vi "DMS_Insert.vi"(4 "Serial No":i32, 7 "DMS":T2, 8 "error in (no error)":errorcluster, 9 "Machine Code":string, 11 "Ref in":T4={"MS SQL Connection"=refnum, "UDL File"=path "", "Time"="", "DCODE"="", "WIP+1"=0, "MC No?"=0, "POKAYOKE?"=FALSE, "Expected Result"="", "Result [Status]"="", "Clock"=0.0, "RFID"="", "WIP Queue"=refnum, "TS Parameter"={"ProfitCenterCode"="", "LineCode"="", "WorkOrderNumber"="", "Model"="", "Model_with_Prefix"="", "VendorCode"="", "SetParameterDateCode"="", "PokaYoke"=0, "Target"=1, "Live_DateCode"="", "CustomerPartNumber"="", "Hand"="", "sBarcode"=FALSE, "FCA"=0, "Ent_Stamp"=timestamp(0 s since 1904-01-01), "STS_CD"=0.0}, "Data_Queue"=[], "RFID Serial No."=""} {"TS Parameter"."FCA" format="%01d"; "TS Parameter"."Target" min=1 max=100000; "TS Parameter"."PokaYoke" min=0 max=1}) -> (0 "error out":errorcluster, 1 "Message":string, 3 "Ref Out":T4={"MS SQL Connection"=refnum, "UDL File"=path "", "Time"="", "DCODE"="", "WIP+1"=0, "MC No?"=0, "POKAYOKE?"=FALSE, "Expected Result"="", "Result [Status]"="", "Clock"=0.0, "RFID"="", "WIP Queue"=refnum, "TS Parameter"={"ProfitCenterCode"="", "LineCode"="", "WorkOrderNumber"="", "Model"="", "Model_with_Prefix"="", "VendorCode"="", "SetParameterDateCode"="", "PokaYoke"=0, "Target"=1, "Live_DateCode"="", "CustomerPartNumber"="", "Hand"="", "sBarcode"=FALSE, "FCA"=0, "Ent_Stamp"=timestamp(0 s since 1904-01-01), "STS_CD"=0.0}, "Data_Queue"=[], "RFID Serial No."=""} {"TS Parameter"."FCA" format="%01d"; "TS Parameter"."Target" min=1 max=100000; "TS Parameter"."PokaYoke" min=0 max=1})   [LabVIEW 2020]
uses:
  Controls/TD SQL.ctl
  <vilib>/addons/database/Connection.llb/Conn ObjectReference.ctl
  Controls/WIP_State.ctl
  Controls/TS_Parameter.ctl
  Controls/DMS_Control.ctl
  Controls/dms_BOOL.ctl
  MS SQL/MS_Global.vi
  <vilib>/addons/database/NI_Database_API.lvlib
panel:
  in  "Machine":T1(ring)
  out "resulting string":string
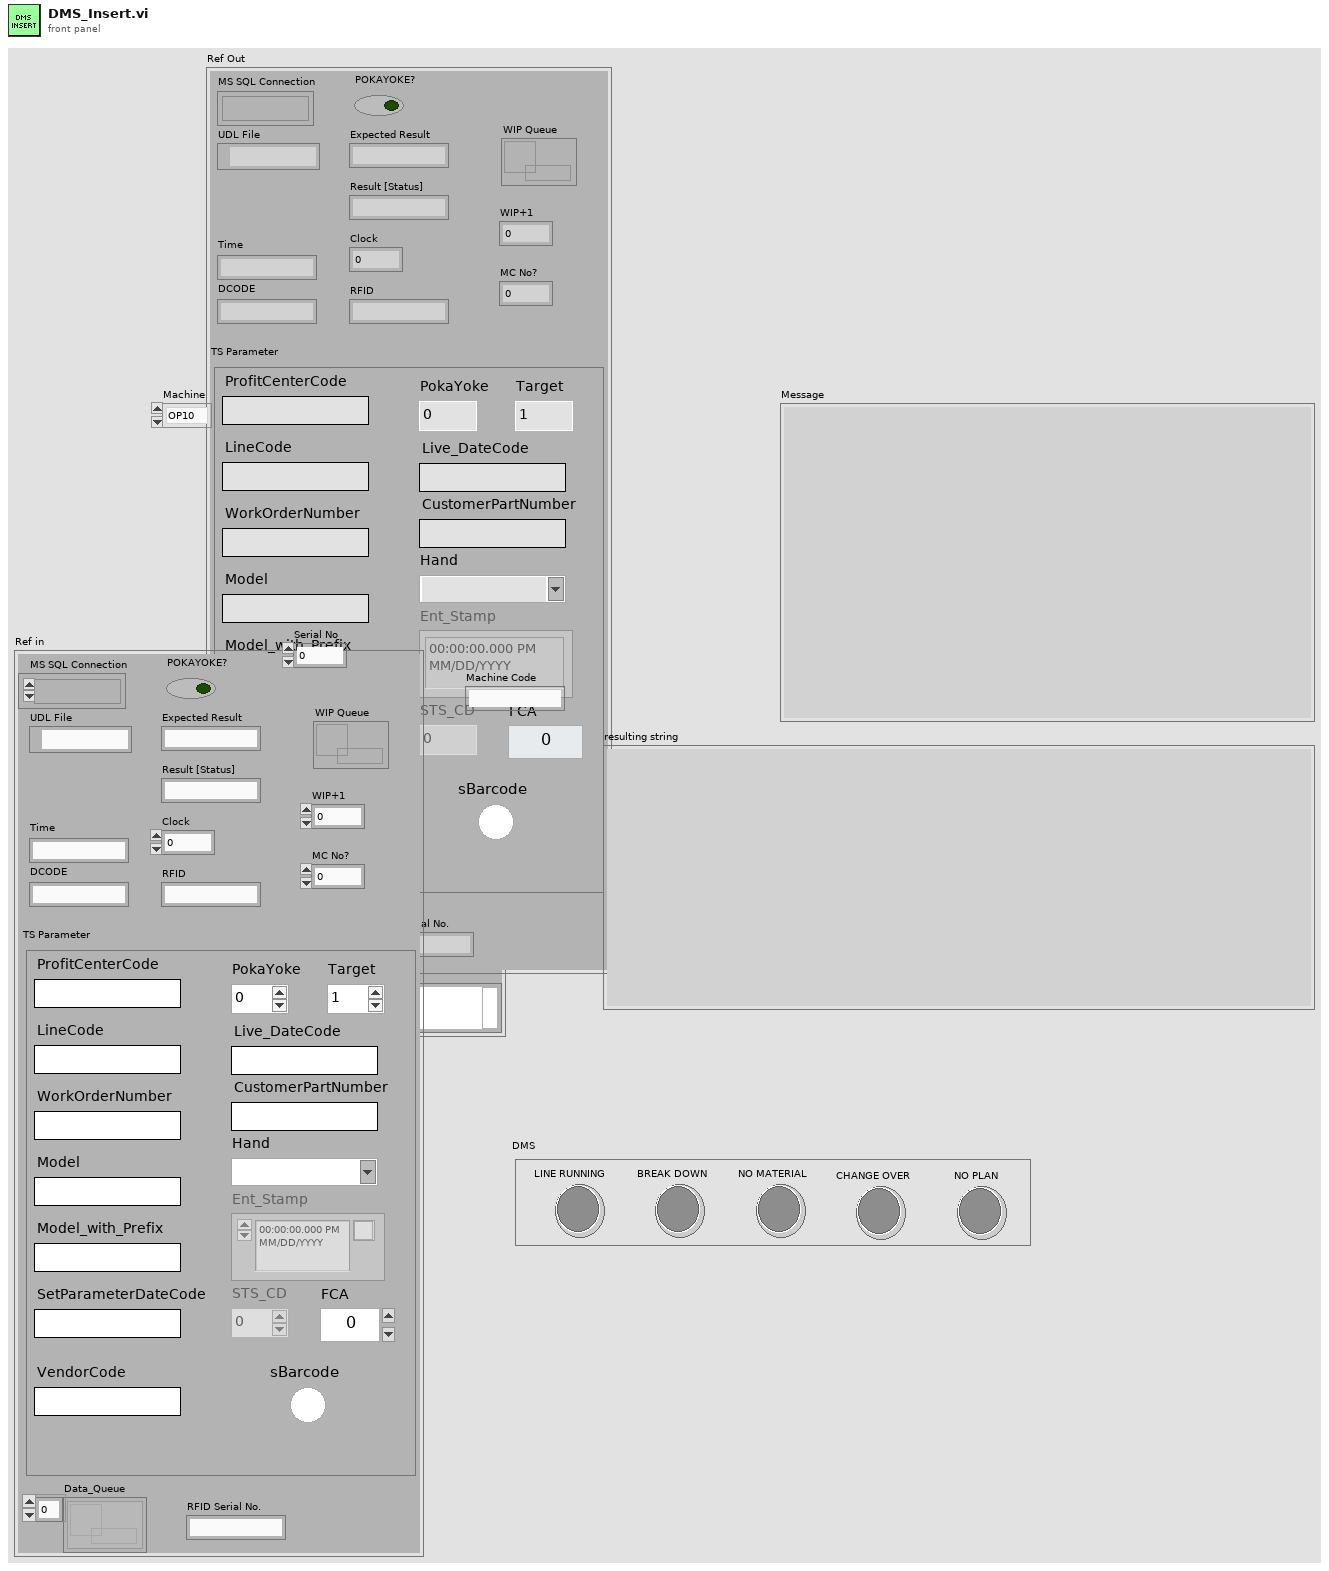
[diagram p1: front panel]
types:
  T1 = enum16{"OP10", "OP20", "OP30", "OP40", "OP50", "OP60", "OP70", "OP80", "LINE"}
  T2 = typedef "DMS_Control.ctl" = cluster{"LINE RUNNING":T3, "BREAK DOWN":T3, "NO MATERIAL":T3, "CHANGE OVER":T3, "NO PLAN":T3}
  T3 = typedef "dms_BOOL.ctl" = bool
  T4 = typedef "TD SQL.ctl" = cluster{"MS SQL Connection":T5, "UDL File":path, "Time":string, "DCODE":string, "WIP+1":i64, "MC No?":i32, "POKAYOKE?":bool, "Expected Result":string, "Result [Status]":string, "Clock":dbl, "RFID":string, "WIP Queue":refnum<queue>, "TS Parameter":T6, "Data_Queue":refnum<queue>[], "RFID Serial No.":string}
  T5 = typedef "NI_Database_API.lvlib/Conn ObjectReference.ctl" = refnum<k1>
  T6 = typedef "TS_Parameter.ctl" = cluster{"ProfitCenterCode":string, "LineCode":string, "WorkOrderNumber":string, "Model":string, "Model_with_Prefix":string, "VendorCode":string, "SetParameterDateCode":string, "PokaYoke":i32, "Target":i32, "Live_DateCode":string, "CustomerPartNumber":string, "Hand":string, "sBarcode":bool, "FCA":i32, "Ent_Stamp":timestamp, "STS_CD":dbl}
  T7 = typedef "Idle_Timer.ctl" = cluster{"OP10":T8, "OP20":T8, "OP30":T8, "OP40":T8, "OP50":T8, "OP60":T8}
  T8 = typedef "Idle_Timer_disp.ctl" = dbl
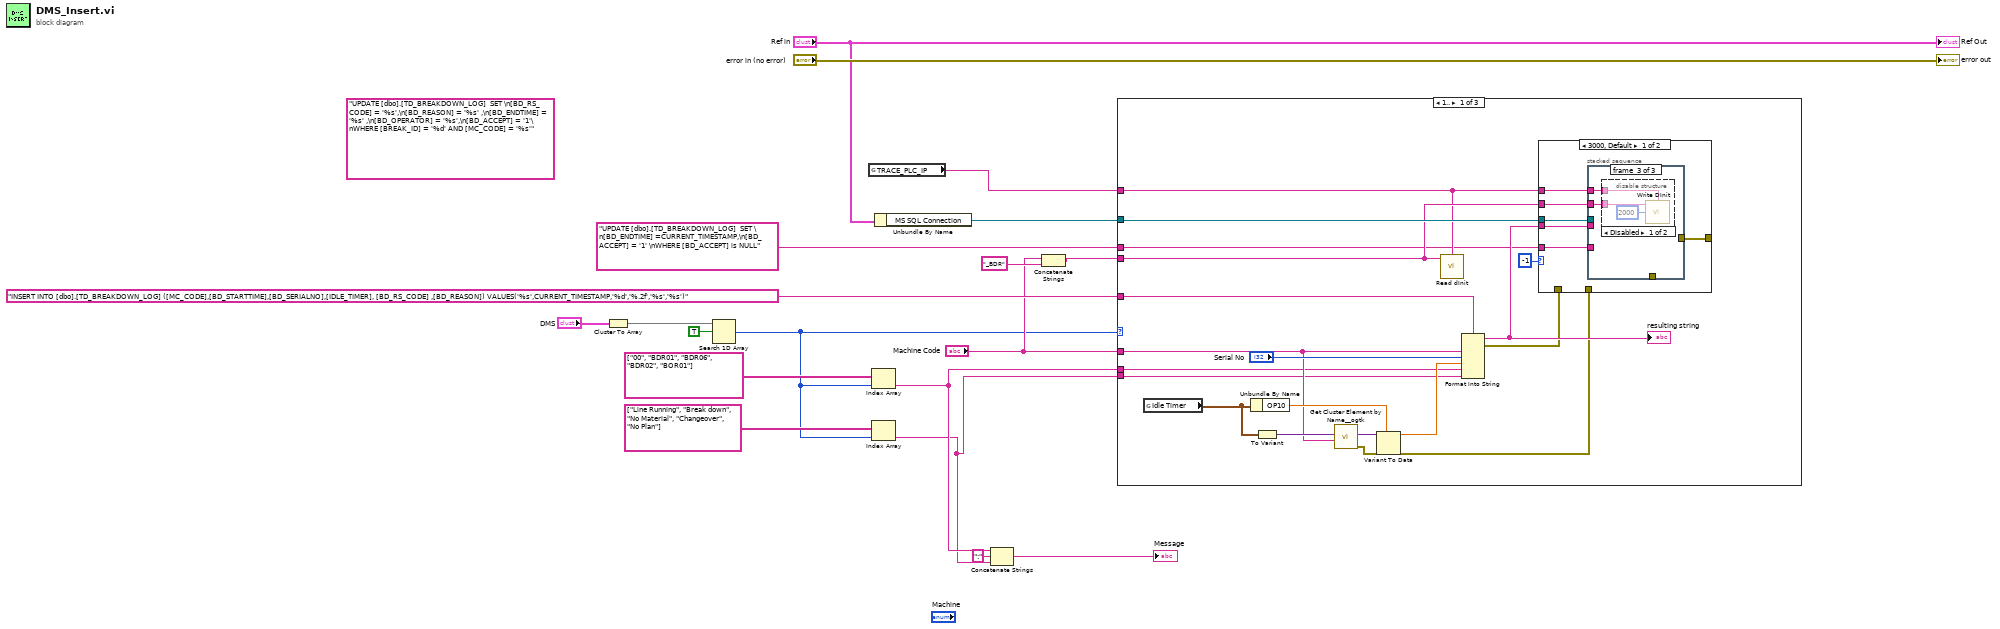
[diagram p0: block diagram]
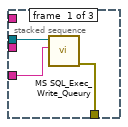
[diagram p2: hidden frame]
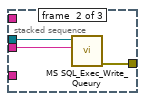
[diagram p3: hidden frame]
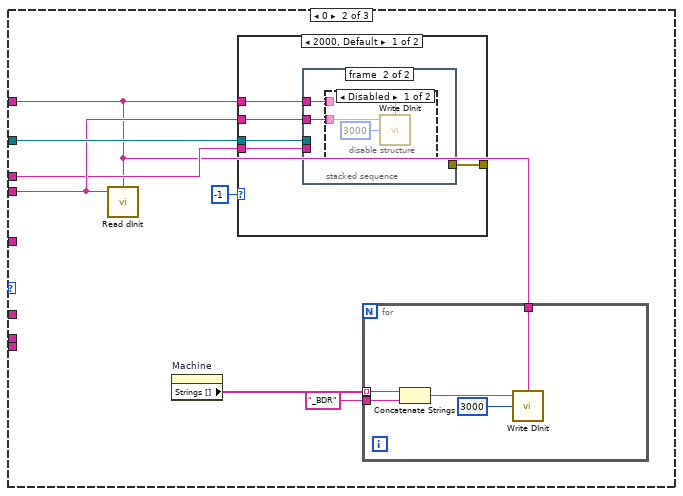
[diagram p6: hidden frame]
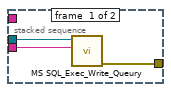
[diagram p7: hidden frame]
diagram:
  (unwired) "UPDATE [dbo].[TD_BREAKDOWN_LOG]  SET \n[BD_RS_CODE] = '%s',\n[BD_REASON] = '%s' ,\n[BD_ENDTIME] = '%s' ,\n[BD_OPERATOR] = '%s',\n[BD_ACCEPT] = '1'\nWHERE [BREAK_ID] = '%d' AND [MC_CODE] = '%s'" ("Operator")
  n1 = Cluster To Array(cluster="DMS") -> (array=w14:T3[])
  n2 = Search 1D Array(1D array=w14, element=TRUE) -> (index of element=w6:i32)  [unwired: 1 in]
  n3 = global read "MS_Global.vi" "TRACE_PLC_IP"() -> (w1:string)
  n4 = Index Array(array=string[] ["00", "BDR01", "BDR06", "BDR02", "BOR01"], index=w6) -> (element=w3:string)
  n5 = Index Array(array=string[] ["Line Running", "Break down", "No Material", "Changeover", "No Plan"], index=w6) -> (element=w2:string)
  n6 = Unbundle By Name("Ref in") -> ("MS SQL Connection"=w17:T5)
  n7 = Concatenate Strings(w3, ":" ("string"), w2) -> (→"Message":string)
  n8 = Concatenate Strings("Machine Code", "_BDR" ("String")) -> (w10:string)
  n9 = case shown="1.." w6 {
    tunnel: w17 -> [w38 w62 _]
    tunnel: "INSERT INTO [dbo].[TD_BREAKDOWN_LOG] ([MC_CODE],[BD_STARTTIME],[BD_SERIALNO],[IDLE_TIMER], [BD_RS_CODE] ,[BD_REASON]) VALUES('%s',CURRENT_TIMESTAMP,'%d','%.2f','%s','%s')" ("Query") -> [w37 _ _]
    tunnel: "Machine Code" -> [w26 _ _]
    tunnel: w10 -> [w25 w61 _]
    tunnel: w1 -> [w24 w58 _]
    tunnel: "UPDATE [dbo].[TD_BREAKDOWN_LOG]  SET \n[BD_ENDTIME] =CURRENT_TIMESTAMP,\n[BD_ACCEPT] = '1' \nWHERE [BD_ACCEPT] is NULL" ("Operator") -> [w20 w60 _]
    tunnel: w3 -> [w23 _ _]
    tunnel: w2 -> [w22 _ _]
    frame 1.. {
      n10 = global read "MS_Global.vi" "Idle Timer"() -> (w33:T7)
      n11 = Unbundle By Name(w33) -> ("OP10"=w29:T8)
      n12 = To Variant(anything=w33) -> (Variant=w32:variant)
      n13 = call <userlib>:"Get Cluster Element by Name__ogtk.vi"("Element Name"=w26, "Cluster"=w32) -> ("error out"=w30:errorcluster, "VElement"=w31:variant)  [unwired: 7 in, 1 out]
      n14 = Variant To Data(error in=w30, type=w29, Variant=w31) -> (data=w28:T8, error out=w27:errorcluster)
      n15 = call "Read dInit.vi"("Network Path"=w24, "Tag Name"=w25) -> ()  [unwired: 3 in, 1 out]
      n16 = Format Into String(format string=w37, w26, "Serial No", w28, w23, w22) -> (resulting string=w36:string, error out=w35:errorcluster)  [unwired: 2 in]
      "resulting string" <- w36
      n17 = case shown="3000, Default" -1 ("Previous Status") {
        tunnel: w38 -> [w44 _]
        tunnel: w36 -> [w43 _]
        tunnel: [w42 _] -> _
        tunnel: w24 -> [w41 _]
        tunnel: w25 -> [w40 _]
        tunnel: w35 -> [_ _]
        tunnel: w27 -> [_ _]
        tunnel: w20 -> [w39 _]
        frame 3000, Default {
          n18 = stacked-sequence {
            tunnel: w44 -> [w46 w50 _]
            tunnel: w43 -> [_ w49 _]
            tunnel: [_ w48 _] -> w42
            tunnel: w41 -> [_ _ w52]
            tunnel: w40 -> [_ _ w51]
            tunnel: w39 -> [w47 _ _]
            tunnel: [w45 _ _] -> _
            frame #0 {
              n19 = call "MS SQL_Exec_Write_Queury.vi"("Query"=w47, "Refnum in"=w46) -> ("error out"=w45:errorcluster)  [unwired: 8 in, 1 out]
            }
            frame #1 {
              n20 = call "MS SQL_Exec_Write_Queury.vi"("Query"=w49, "Refnum in"=w50) -> ("error out"=w48:errorcluster)  [unwired: 8 in, 1 out]
            }
            frame #2 {
              n21 = disable-structure shown="Disabled" {
                disable-tunnel: w52 -> [w55 _]
                disable-tunnel: w51 -> [w54 _]
                frame Disabled {
                  n22 = call "Write DInit.vi"("Network Path"=w55, "Int"=2000, "Tag Name"=w54) -> ()  [unwired: 2 in]
                }
                frame Enabled {
                }
              }
            }
          }
        }
        frame 2000 {
        }
      }
    }
    frame 0 {
      n23 = call "Read dInit.vi"("Network Path"=w58, "Tag Name"=w61) -> ()  [unwired: 3 in, 1 out]
      n24 = property on="Machine" class="Enum (strict)"() -> ("Strings []"=w57:string[])  [unwired: 2 in, 2 out]
      n25 = case shown="2000, Default" -1 ("Previous Status") {
        tunnel: w62 -> [w72 _]
        tunnel: w60 -> [w71 _]
        tunnel: [w70 _] -> _
        tunnel: w58 -> [w69 _]
        tunnel: w61 -> [w68 _]
        frame 2000, Default {
          n26 = stacked-sequence {
            tunnel: w72 -> [w75 _]
            tunnel: w71 -> [w74 _]
            tunnel: [w73 _] -> w70
            tunnel: w69 -> [_ w77]
            tunnel: w68 -> [_ w76]
            frame #0 {
              n27 = call "MS SQL_Exec_Write_Queury.vi"("Query"=w74, "Refnum in"=w75) -> ("error out"=w73:errorcluster)  [unwired: 8 in, 1 out]
            }
            frame #1 {
              n28 = disable-structure shown="Disabled" {
                disable-tunnel: w77 -> [w80 _]
                disable-tunnel: w76 -> [w79 _]
                frame Disabled {
                  n29 = call "Write DInit.vi"("Network Path"=w80, "Int"=3000, "Tag Name"=w79) -> ()  [unwired: 2 in]
                }
                frame Enabled {
                }
              }
            }
          }
        }
        frame 3000 {
        }
      }
      n30 = for {
        tunnel: w58 -> [w66]
        tunnel: w57 -> [w65] mode=indexing
        tunnel: "_BDR" ("String") -> [w64]
        n31 = Concatenate Strings(w65, w64) -> (w63:string)
        n32 = call "Write DInit.vi"("Network Path"=w66, "Int"=3000, "Tag Name"=w63) -> ()  [unwired: 2 in]
      }
    }
    frame -1, Default {
    }
  }
  "error out" <- "error in (no error)"
  "Ref Out" <- "Ref in"
